vi "4155C Config SMU.vi"(0 "VISA session":refnum<visa-resource-name>, 1 "I name (max 6 chars)":string, 2 "Range mode":u16(ring) items=["Auto", "Limited", "Fixed"], 3 "series resistance *":u32(slide) max=3 scale=0.0..3.0, 5 "unit to configure":u32(slide) max=5 scale=0.0..5.0, 9 "function":u32(slide) max=4 scale=0.0..4.0, 10 "standby":bool, 11 "error in (no error)":errorcluster, 12 "V name (max 6 chars)":string, 13 "Range":u8(slide)=6 max=11 scale=0.0..11.0, 14 "mode":u32(slide) max=4 scale=0.0..4.0) -> (4 "dup VISA resource name":refnum<visa-resource-name>, 15 "error out":errorcluster)   [LabVIEW 2019]
doc: "This VI configures an SMU for SWEEP mode measurement. \n\nThis VI corresponds to the Channel Definition Page of the instrument (when Measurement Mode is SWEEP). In general, it allows every setting change that can be made via the instrument's front panel although the change may cause a setting conflict when a measurement is initialied. This VI doesnot allow (by reporting an error) setting changes that can not be made via the instrument's front panel. For example, you may not set Series Resistance for units other than SMU1, SMU2/5.\n\n** The instrument used in the development of this instrument driver does not have an Expander Unit installed. Therefore commands related to SMU5/6 have not been verified."
panel:
  # "<--->"
  # "*   The Series Resistance control is active only if UnitToConfigure is SMU1 or SMU2/SMU5 (see description)\n** This VI does NOT report all setting errors.  Error checking must be done when a measurement is initialized."
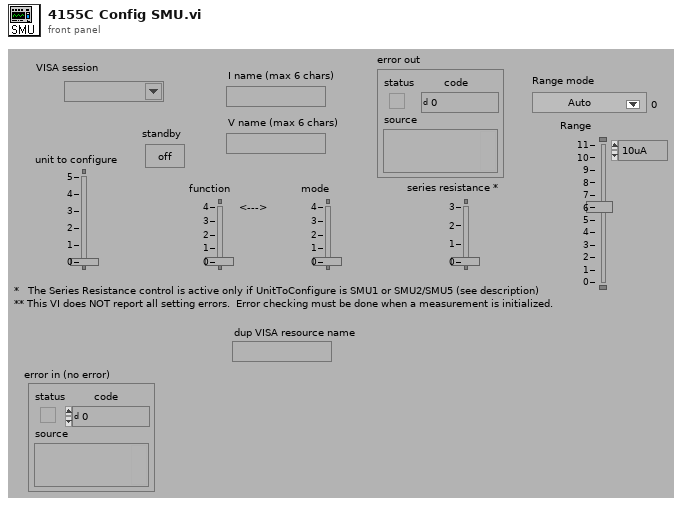
[diagram p1: front panel]
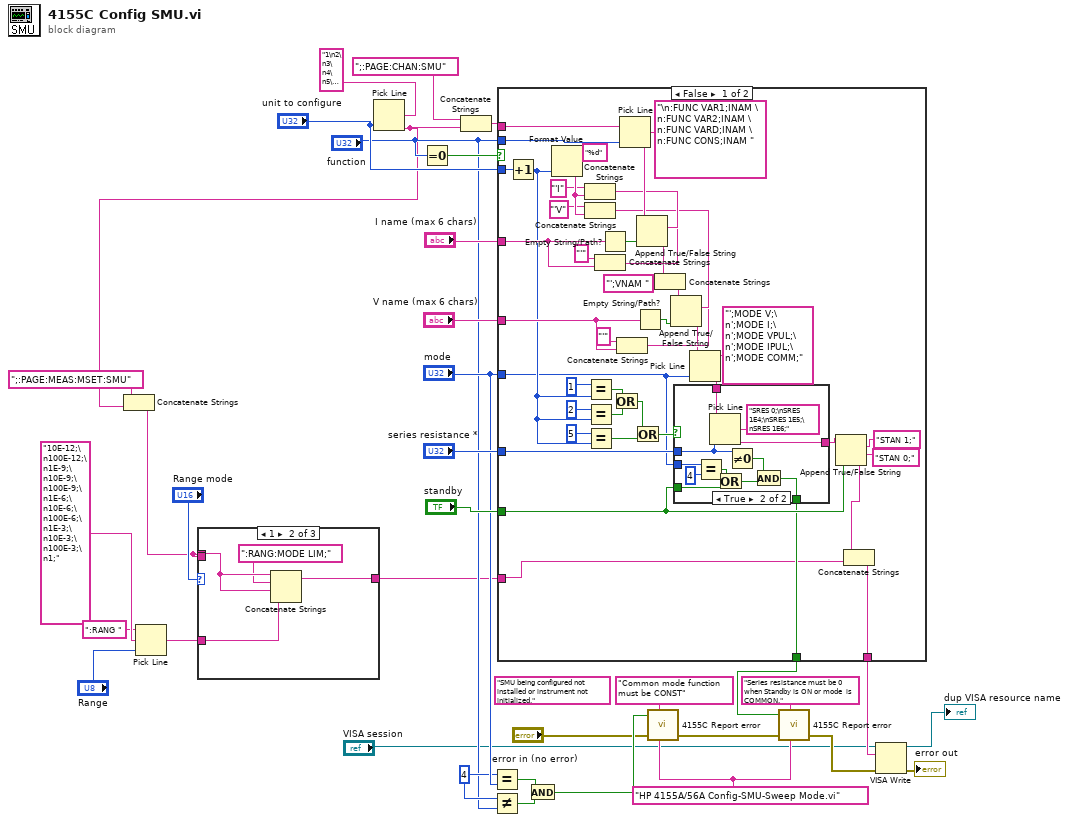
[diagram p0: block diagram]
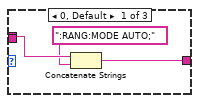
[diagram p2: hidden frame]
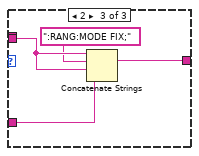
[diagram p3: hidden frame]
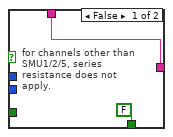
[diagram p4: hidden frame]
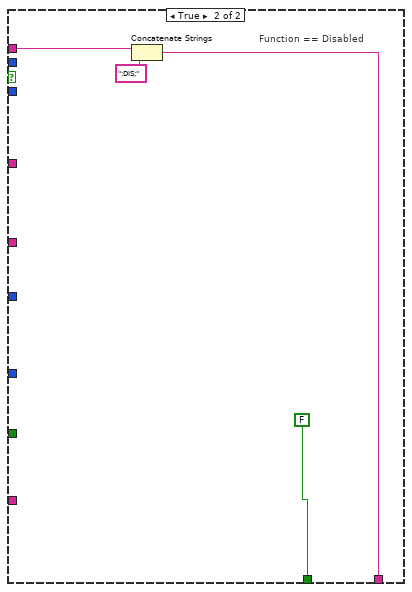
[diagram p5: hidden frame]
diagram:
  w22 = 4
  (unwired) "SMU being configured not installed or instrument not initialized."
  w15 = "HP 4155A/56A Config-SMU-Sweep Mode.vi"
  n1 = Pick Line(string ("")=":RANG ", multi-line string="10E-12;\n100E-12;\n1E-9;\n10E-9;\n100E-9;\n1E-6;\n10E-6;\n100E-6;\n1E-3;\n10E-3;\n100E-3;\n1;", line index="Range") -> (output string=w6:string)
  n2 = Pick Line(multi-line string="1\n2\n3\n4\n5\n6", line index="unit to configure") -> (output string=w3:string)  [unwired: 1 in]
  n3 = Concatenate Strings(";:PAGE:MEAS:MSET:SMU" ("Substring"), w3) -> (w1:string)
  n4 = case shown="1" "Range mode" {
    tunnel: w6 -> [_ w42 w44]
    tunnel: [w36 w39 w45] -> w5
    tunnel: w1 -> [w38 w41 _]
    tunnel: w1 -> [_ _ w46]
    frame 0, Default {
      n5 = Concatenate Strings(w38, ":RANG:MODE AUTO;" ("multi-line string")) -> (w36:string)
    }
    frame 1 {
      n6 = Concatenate Strings(w41, ":RANG:MODE LIM;" ("multi-line string"), w41, w42) -> (w39:string)
    }
    frame 2 {
      n7 = Concatenate Strings(w46, ":RANG:MODE FIX;" ("multi-line string"), w46, w44) -> (w45:string)
    }
  }
  n8 = Equal To 0?(x="function") -> (x = 0?=w29:bool)
  n9 = Concatenate Strings(";:PAGE:CHAN:SMU", w3) -> (w9:string)
  n10 = Equal?(x=w22, y="mode") -> (x = y?=w26:bool)
  n11 = Not Equal?(x=w22, y="function") -> (x != y?=w25:bool)
  n12 = case shown="False" w29 {
    tunnel: w9 -> [w48 w107]
    tunnel: "function" -> [w87 _]
    tunnel: "unit to configure" -> [w56 _]
    tunnel: "I name (max 6 chars)" -> [w81 _]
    tunnel: "V name (max 6 chars)" -> [w72 _]
    tunnel: "mode" -> [w52 _]
    tunnel: "series resistance *" -> [w65 _]
    tunnel: "standby" -> [w53 _]
    tunnel: [w49 w105] -> w31
    tunnel: [w51 FALSE] -> w17
    tunnel: w5 -> [w47 _]
    frame False {
      n13 = Increment(x=w56) -> (x+1=w54:u32)
      n14 = Format Value(format string="%d", value (0)=w54) -> (output string=w85:string)  [unwired: 1 in]
      n15 = Concatenate Strings("'I", w85) -> (w82:string)
      n16 = Concatenate Strings("'V", w85) -> (w75:string)
      n17 = Equal?(x=1, y=w54) -> (x = y?=w61:bool)
      n18 = Equal?(x=2, y=w54) -> (x = y?=w60:bool)
      n19 = Equal?(x=5, y=w54) -> (x = y?=w59:bool)
      n20 = Concatenate Strings("'", w81) -> (w79:string)
      n21 = Empty String/Path?(string/path=w81) -> (empty?=w88:bool)
      n22 = Or(x=w61, y=w60) -> (x .or. y?=w58:bool)
      n23 = Concatenate Strings("'", w72) -> (w71:string)
      n24 = Pick Line(string ("")=w48, multi-line string="\n:FUNC VAR1;INAM \n:FUNC VAR2;INAM \n:FUNC VARD;INAM \n:FUNC CONS;INAM ", line index=w87) -> (output string=w89:string)
      n25 = Or(x=w58, y=w59) -> (x .or. y?=w57:bool)
      n26 = Empty String/Path?(string/path=w72) -> (empty?=w74:bool)
      n27 = Append True/False String(1:w88, 2:w79, 3:w82, 4:w89) -> (0:w78:string)
      n28 = Concatenate Strings(w78, "';VNAM ") -> (w76:string)
      n29 = Append True/False String(1:w74, 2:w71, 3:w75, 4:w76) -> (0:w69:string)
      n30 = Pick Line(string ("")=w69, multi-line string="';MODE V;\n';MODE I;\n';MODE VPUL;\n';MODE IPUL;\n';MODE COMM;", line index=w52) -> (output string=w66:string)
      n31 = case shown="True" w57 {
        tunnel: w66 -> [w92 w102]
        tunnel: w65 -> [_ w95]
        tunnel: [w92 w101] -> w64
        tunnel: w53 -> [_ w98]
        tunnel: w52 -> [_ w100]
        tunnel: [FALSE w93] -> w51
        frame False {
          # "for channels other than\nSMU1/2/5, series \nresistance does not \napply."
        }
        frame True {
          n32 = Equal?(x=w100, y=4) -> (x = y?=w97:bool)
          n33 = Pick Line(string ("")=w102, multi-line string="SRES 0;\nSRES 1E4;\nSRES 1E5;\nSRES 1E6;", line index=w95) -> (output string=w101:string)
          n34 = Or(x=w97, y=w98) -> (x .or. y?=w96:bool)
          n35 = Not Equal To 0?(x=w95) -> (x != 0?=w94:bool)
          n36 = And(x=w94, y=w96) -> (x .and. y?=w93:bool)
        }
      }
      n37 = Append True/False String(1:w53, 2:"STAN 0;", 3:"STAN 1;", 4:w64) -> (0:w50:string)
      n38 = Concatenate Strings(w50, w47) -> (w49:string)
    }
    frame True {
      # "Function == Disabled"
      n39 = Concatenate Strings(w107, ":DIS;") -> (w105:string)
    }
  }
  n40 = And(x=w26, y=w25) -> (x .and. y?=w24:bool)
  n41 = call "4155C Report error.vi"("new error"=w24, "error message"="Common mode function must be CONST", "error in (no error)"="error in (no error)", "source"=w15) -> ("error out"=w19:errorcluster)  [unwired: 1 in]
  n42 = call "4155C Report error.vi"("new error"=w17, "error message"="Series resistance must be 0 when Standby is ON or mode  is COMMON.", "error in (no error)"=w19, "source"=w15) -> ("error out"=w16:errorcluster)  [unwired: 1 in]
  n43 = VISA Write(VISA resource name="VISA session", write buffer=w31, error in (no error)=w16) -> (VISA resource name out=→"dup VISA resource name":refnum<visa-resource-name>, error out=→"error out":errorcluster)  [unwired: 1 out]
